vi "network_stream_reader.vi"() -> ()   [LabVIEW 2017]
uses:
  diode_charts.ctl
  <vilib>/dex/Stream Element Allocation Mode.ctl
panel:
  out "data out":T1
  in  "stop":bool
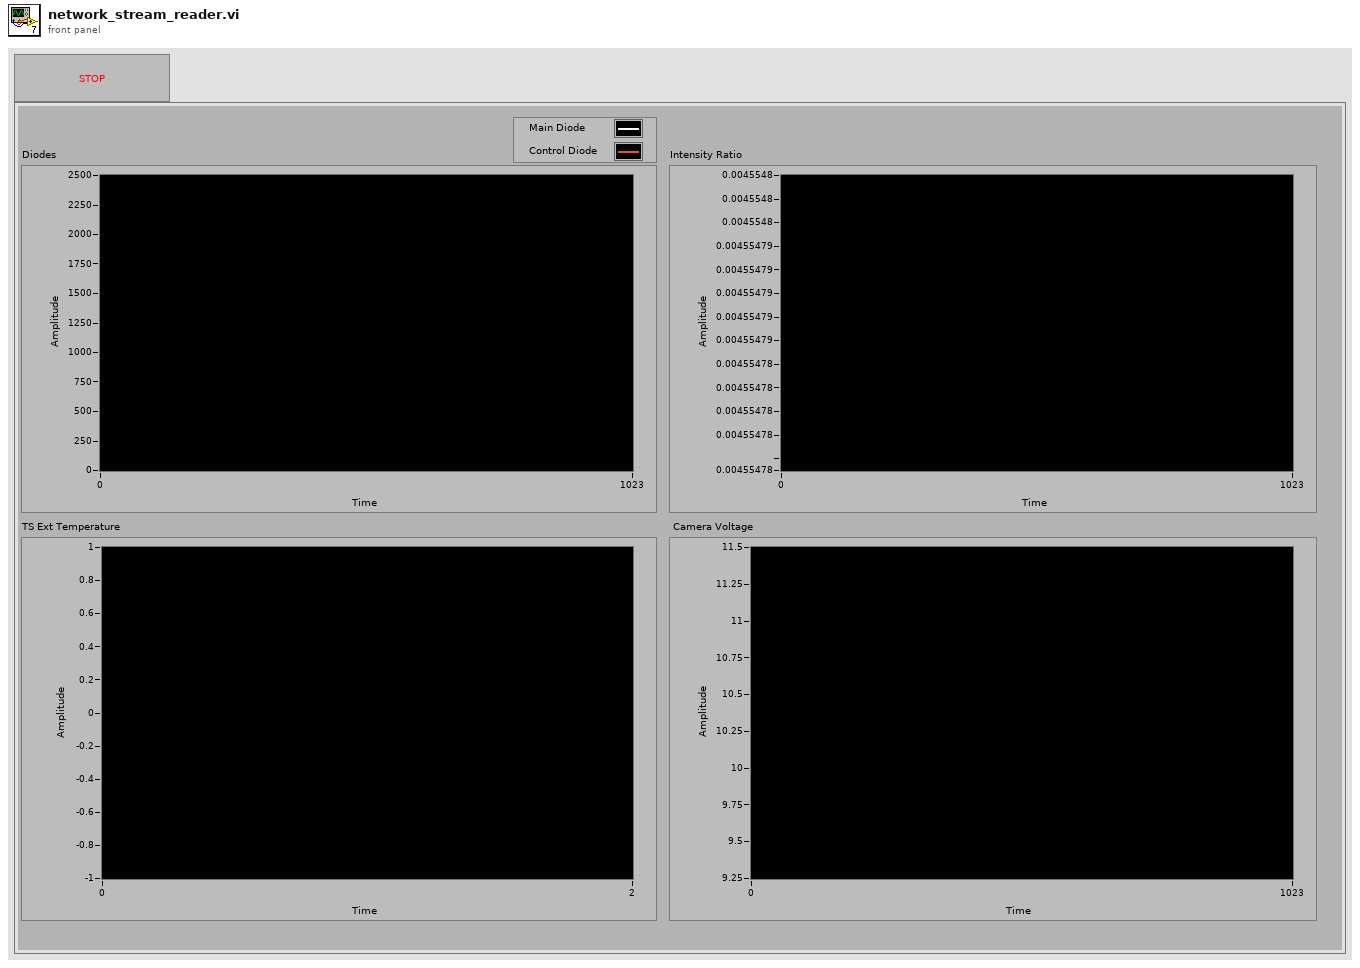
[diagram p1: front panel]
types:
  T1 = typedef "diode_charts.ctl" = cluster{"Diodes":cluster{dbl, dbl}[], "Intensity Ratio":dbl[], "TS Ext Temperature":dbl[], " Camera Voltage":dbl[]}
  T2 = typedef "Stream Element Allocation Mode.ctl" = u32
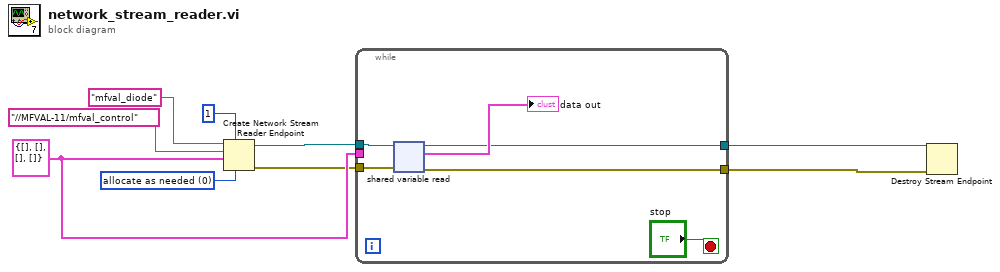
[diagram p0: block diagram]
diagram:
  w2 = T2 0 items=["allocate as needed", "pre-allocate"] ("element allocation mode")
  w9 = T1 {"Diodes"=[], "Intensity Ratio"=[], "TS Ext Temperature"=[], " Camera Voltage"=[]} ("Diode Charts")
  n1 = Create Network Stream Reader Endpoint(6:w2, 7:1 ("writer buffer size"), 9:w9, 10:"//MFVAL-11/mfval_control" ("writer url"), 11:"mfval_diode" ("writer name")) -> (0:w8:errorcluster, 3:w4:refnum<k21>)  [unwired: 2 in]
  n2 = while {
    tunnel: w9 -> [_]
    tunnel: w8 -> [w14]
    tunnel: [w13] -> w6
    tunnel: [w11] -> w5
    tunnel: w4 -> [w10]
    stop <- "stop" stop-if-true
    n3 = shared-variable-read(w10, w14) -> (w11:refnum<k21>, w13:errorcluster, →"data out":T1)  [unwired: 1 in, 1 out]
  }
  n4 = Destroy Stream Endpoint(8:w6, 11:w5) -> ()  [unwired: 1 out]
